vi "Main.vi"() -> ()   [LabVIEW 2019, in "Server.lvlib"]
doc: "This template is based off of the Queued Message Handler design pattern and the Queued Message Handler project template that ships with LabVIEW.\n\nThe main difference is that the queue is private to this module and communication between modules is performed via Broadcast and Request events.\n\nRequest events are wrapped in public API methods and are handled in the Event Handling Loop (EHL) of this VI. Any module can register for Broadcast events sent by this module. The EHL generates messages based on user interface actions.\n\nThe Message Handling Loop (MHL) processes messages generated by the EHL, or by other messages. The messages are string values, so new messages can be added easily to the Message Cases case structure in the MHL. Each message cluster can also provide an optional value for Message Data, which is a variant that can be converted to whatever message-specific data is required.\n_____\nBased on Delacor QMH Project Template 4.2.1.64."
uses:
  Server.lvlib
  <vilib>/Delacor/Delacor QMH/Libraries/Module Admin_class/Delacor_lib_QMH_Module Admin.lvclass
  TypeDef/ISO.ctl
  TypeDef/Link.ctl
  TypeDef/Noise.ctl
  Module Data--cluster.ctl
  Do Something Argument--cluster.ctl
  <vilib>/Delacor/Delacor QMH/Libraries/Message Queue_class/Delacor_lib_QMH_Message Queue.lvclass/Delacor_lib_QMH_Message Queue.ctl
  Do Something Else Argument--cluster.ctl
  Do Something Else and Wait for Reply Argument--cluster.ctl
  Do Something Else and Wait (Reply Payload)--cluster.ctl
  Stop Argument--cluster.ctl
  TypeDef/Sett data.ctl
  Update control Argument--cluster.ctl
  <vilib>/Delacor/Delacor QMH/Libraries/Module Admin_class/Delacor_lib_QMH_Module Admin.lvclass/Delacor_lib_QMH_Module Admin.ctl
  TypeDef/Analys data.ctl
  TypeDef/Analys type.ctl
  <vilib>/Delacor/Delacor QMH/Libraries/Message Queue_class/Delacor_lib_QMH_Enqueue Message (Single).vi
  <vilib>/Delacor/Delacor QMH/Libraries/Module Admin_class/Delacor_lib_QMH_Get External Launch.vi
  <vilib>/Utility/error.llb/Error Cluster From Error Code.vi
  <vilib>/ErrorRing/Error Ring.xnode
  <vilib>/Delacor/Delacor QMH/Libraries/Message Queue_class/Delacor_lib_QMH_Message Queue.lvclass
  Interrogator/DOWNLINK.lvlib
  UPLINK/UPLINK.lvlib
  Setting Panel/Setting Panel.lvlib
panel:
  in  "Tab Control":enum32{"Main", "Setting"}(tab)
  in  "Иммитатор расстояния":dbl(slide)=3.0 min=3.0 max=1500.0 step=1.0 scale=3.0..1500.0
  in  "Усилитель сигнала":dbl(knob)=1.0 min=1.0 max=100.0 step=1.0 scale=1.0..30.0
  in  "Выбор стандарта":T1
  in  "Аттенюатор шума":dbl(knob)=1.0 min=1.0 max=10.0 step=0.1 scale=1.0..30.0
  in  "Bit rate":dbl=32.0 min=4.0 max=128.0 step=4.0
  in  "Filter":i32=3 min=1 max=15 step=1
  in  "Type noise w":T2
  in  "M w":cluster{"Метка":i64, "Считыветель":i64}={"Метка"=10, "Считыветель"=100} {"Считыветель" min=10 max=10 step=100; "Метка" min=10 max=10 step=100}
  in  "BM":cluster{"R":dbl, "C":dbl, "L":dbl}={"R"=1.0, "C"=0.01, "L"=1e-05} {"L" min=1e-05 max=1.5e-05 step=1e-06 format="%#_6p"; "C" min=0.01 max=0.15 step=0.001 format="%#_6p"; "R" min=1.0 max=150.0 step=1.0 format="%#_6p"}
  in  "BI":cluster{"R":dbl, "C":dbl, "L":dbl}={"R"=1.0, "C"=0.01, "L"=1e-05} {"L" min=1e-05 max=1.5e-05 step=1e-06 format="%#_6p"; "C" min=0.01 max=0.15 step=0.001 format="%#_6p"; "R" min=1.0 max=150.0 step=1.0 format="%#_6p"}
  in  "Apply":bool
  in  "Shutdown":bool
  in  "Link":T3
  in  "Simulate MHL Error":bool
  in  "Simulate EHL Error":bool
  out "error out":errorcluster
  in  "Module Admin":refnum<class "Delacor_lib_QMH_Module Admin.lvclass">
  out "X":dbl
  out "Status":string
  in  "Do Something Else <Replace Me>":bool
  in  "Do Something <Replace Me>":bool
  # "Настройки"
  # "мм"
  # "БУПУЭМСС"
  # "БУПУЭМСМ"
  # "Коэффициент модуляции, %"
  # "Порядок фильтра"
  # "Скорость"
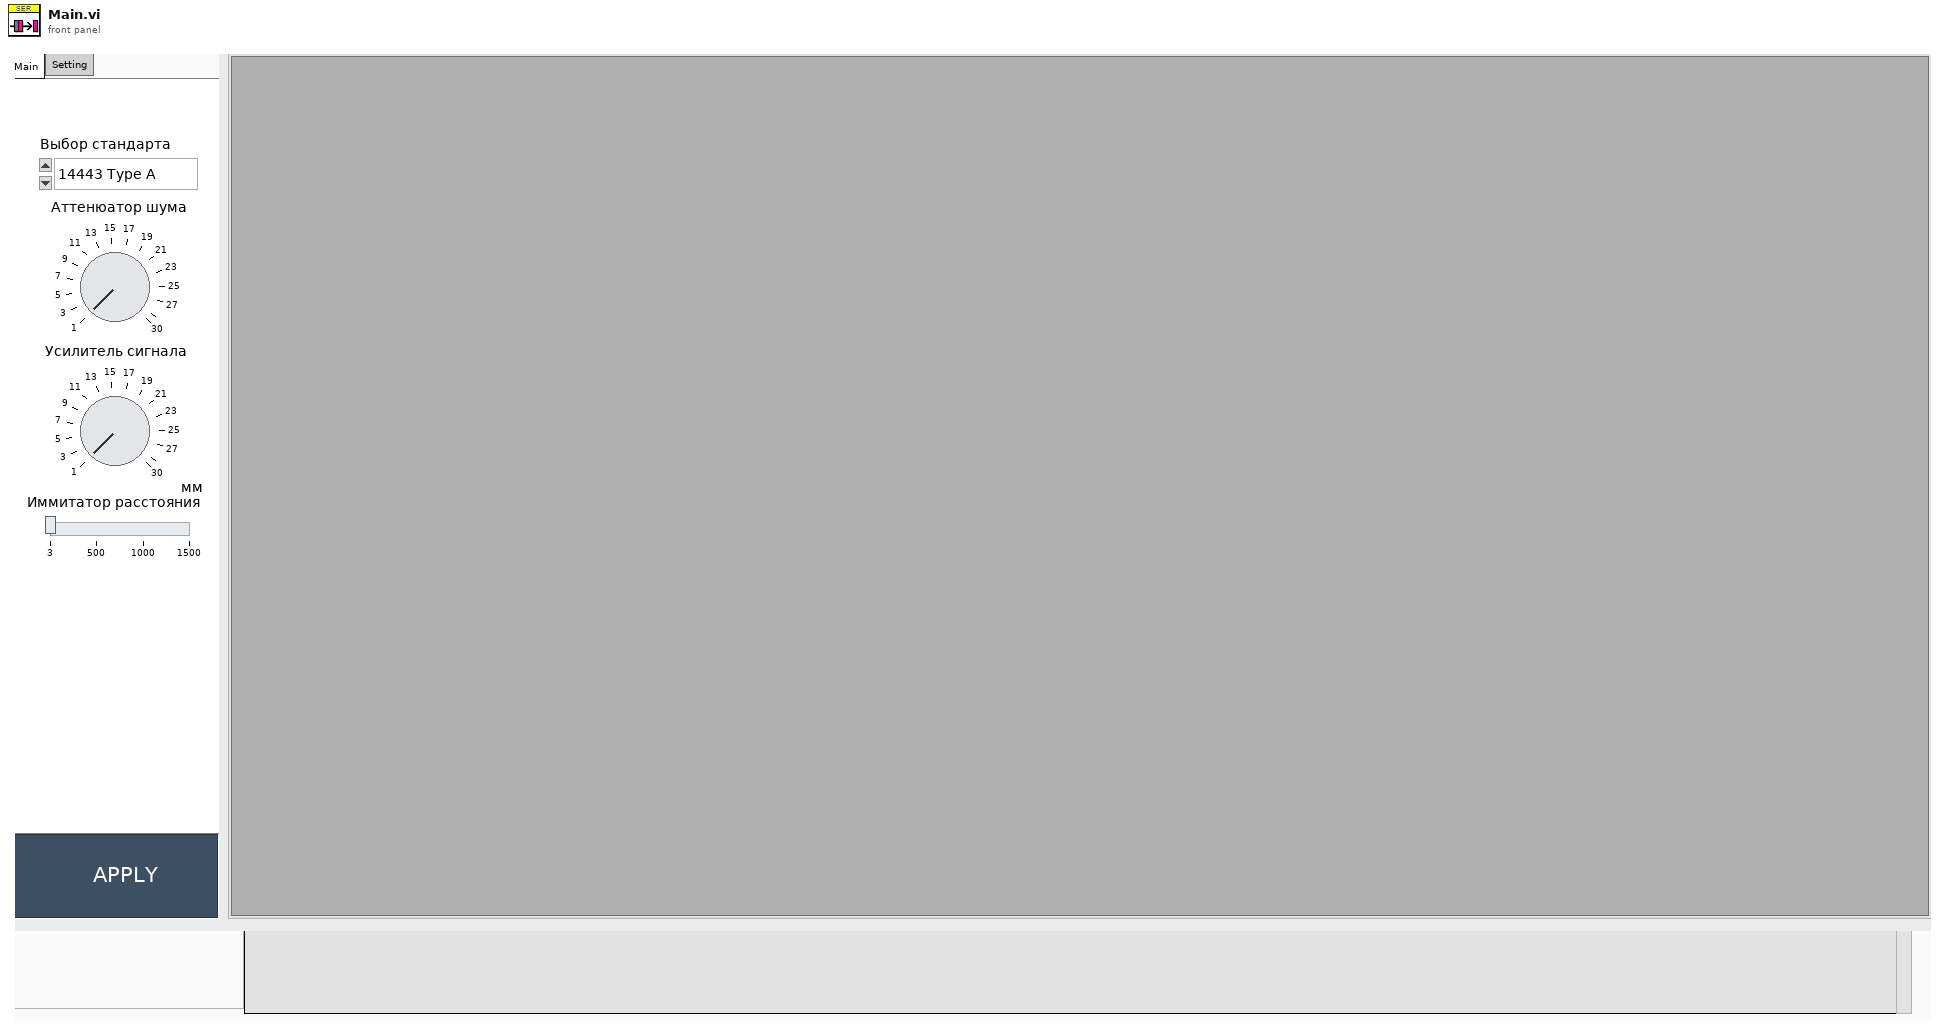
[diagram p1: front panel]
types:
  T1 = typedef "ISO.ctl" = enum16{"14443 Type A", "14443 Type B", "Felica", "15693"}
  T2 = typedef "Noise.ctl" = enum16{"Гауссовский шум", "Белый шум"}
  T3 = typedef "Link.ctl" = enum16{"UPLINK", "DOWNLINK"}
  T4 = typedef "Server.lvlib/Request Events--cluster.ctl" = cluster{"Stop Module":refnum<user-event>, "Do Something":refnum<user-event>, "Do Something Else":refnum<user-event>, "Do Something Else and Wait for Reply":refnum<user-event>, "Show Panel":refnum<user-event>, "Hide Panel":refnum<user-event>, "Get Module Execution Status":refnum<user-event>, "Show Diagram":refnum<user-event>, "Update control":refnum<user-event>}
  T5 = typedef "UPLINK.lvlib/Broadcast Events--cluster.ctl" = cluster{"Module Did Init":refnum<user-event>, "Status Updated":refnum<user-event>, "Error Reported":refnum<user-event>, "Did Something":refnum<user-event>, "Module Did Stop":refnum<user-event>, "Update Module Execution Status":refnum<user-event>}
  T6 = typedef "DOWNLINK.lvlib/Broadcast Events--cluster.ctl" = cluster{"Module Did Init":refnum<user-event>, "Status Updated":refnum<user-event>, "Error Reported":refnum<user-event>, "Did Something":refnum<user-event>, "Module Did Stop":refnum<user-event>, "Update Module Execution Status":refnum<user-event>}
  T7 = typedef "Setting Panel.lvlib/Broadcast Events--cluster.ctl" = cluster{"Module Did Init":refnum<user-event>, "Status Updated":refnum<user-event>, "Error Reported":refnum<user-event>, "Did Something":refnum<user-event>, "Module Did Stop":refnum<user-event>, "Update Module Execution Status":refnum<user-event>, "Get data":refnum<user-event>}
  T8 = typedef "Server.lvlib/Module Data--cluster.ctl" = cluster{"Status":string}
  T9 = typedef "Server.lvlib/Do Something Argument--cluster.ctl" = cluster{"Do Something Msg":string}
  T10 = typedef "Server.lvlib/Do Something Else Argument--cluster.ctl" = cluster{"Do Something Else Msg":string, "X":dbl}
  T11 = typedef "Server.lvlib/Do Something Else and Wait for Reply Argument--cluster.ctl" = cluster{"Do Something Else Msg":string, "X":dbl, "Wait Notifier":refnum<notifier>, "wait for reply":bool}
  T12 = enum32{"invalid lock state", "Not Locked", "Locked (No Password)", "Password-protected"}
  T13 = typedef "Server.lvlib/Stop Argument--cluster.ctl" = cluster{"Origin":string, "Exit via Stop Module Req?":bool, "Wait for Module to stop?":bool}
  T14 = typedef "Sett data.ctl" = cluster{"Filter":i32, "Gain":dbl, "Bit rate":dbl, "ISO/IEC w ":T1, "BI":cluster{"R":dbl, "C":dbl, "L":dbl}, "BM":cluster{"R":dbl, "C":dbl, "L":dbl}, "M":cluster{"Метка":i64, "Считыветель":i64}, "Type noise":T2, "Link":T3, "Noise attenuator":dbl, "Signal gain":dbl, "Distance":dbl}
  T15 = enum8{"Enabled", "Disabled", "Disabled and Grayed Out"}
  T16 = typedef "Server.lvlib/Update control Argument--cluster.ctl" = cluster{"Variant":variant}
  T17 = enum32{"Invalid", "Standard", "Closed", "Hidden", "Minimized", "Maximized"}
  T18 = typedef "Server.lvlib/Do Something Else and Wait (Reply Payload)--cluster.ctl" = cluster{"Value":dbl, "error":errorcluster}
  T19 = typedef "Analys data.ctl" = cluster{"min attenuator":dbl, "max distanse":dbl, "num sample":dbl, "type":T20}
  T20 = typedef "Analys type.ctl" = enum16{"Noise", "Distance"}
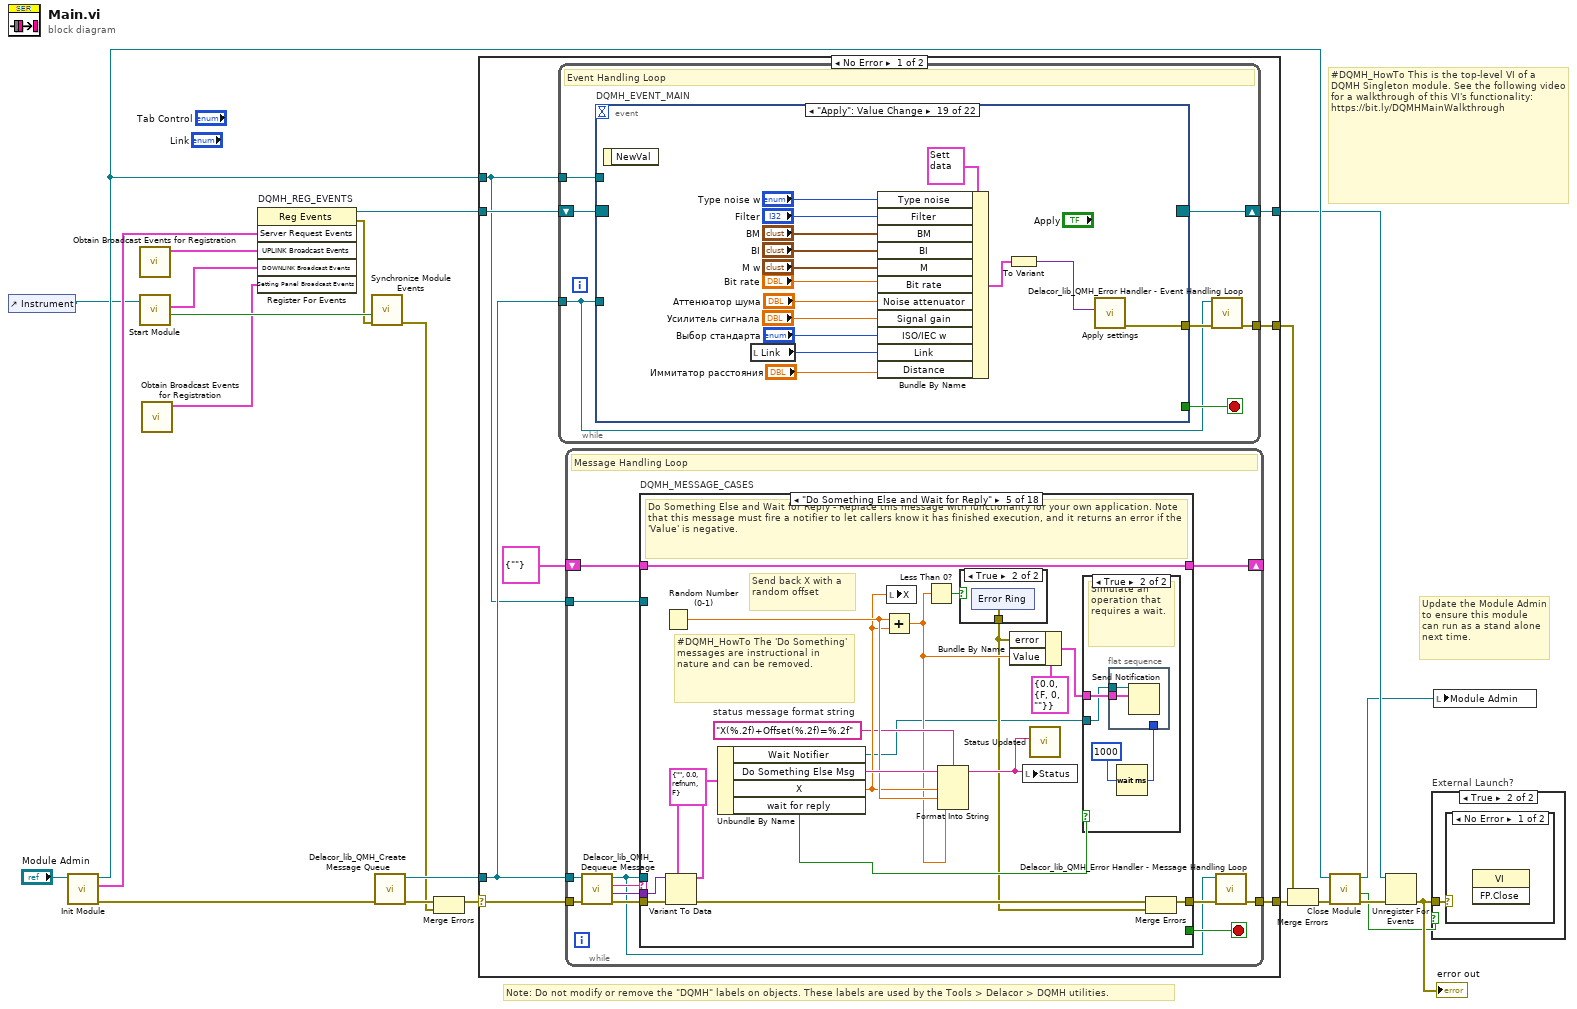
[diagram p0: block diagram]
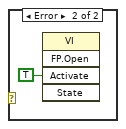
[diagram p3: hidden frame]
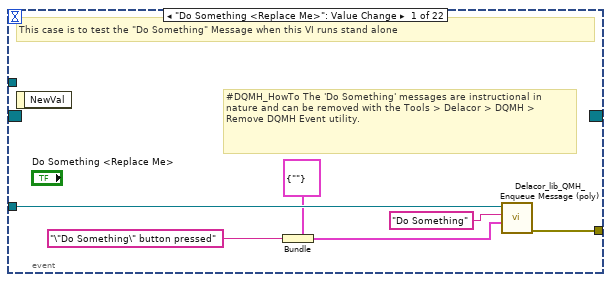
[diagram p4: hidden frame]
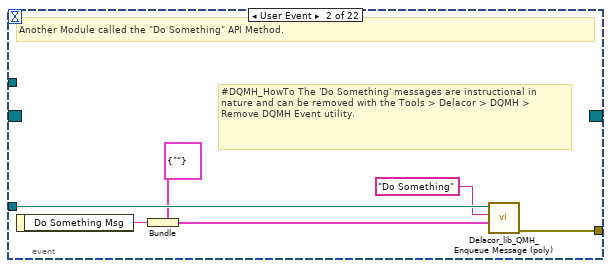
[diagram p5: hidden frame]
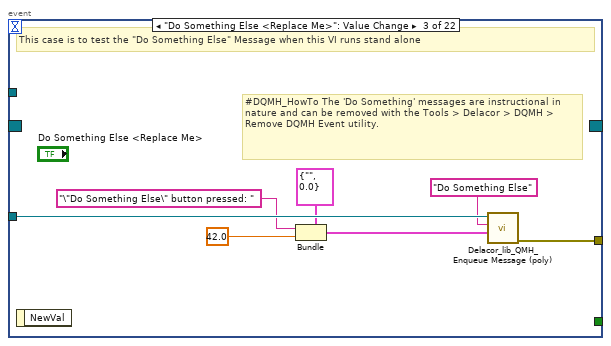
[diagram p6: hidden frame]
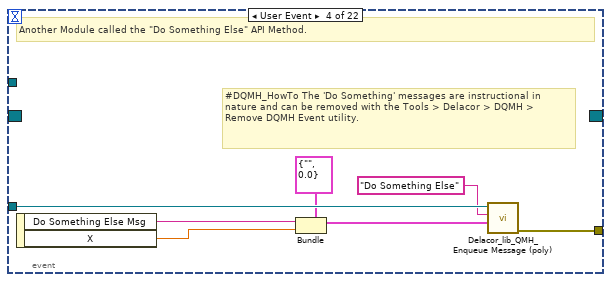
[diagram p7: hidden frame]
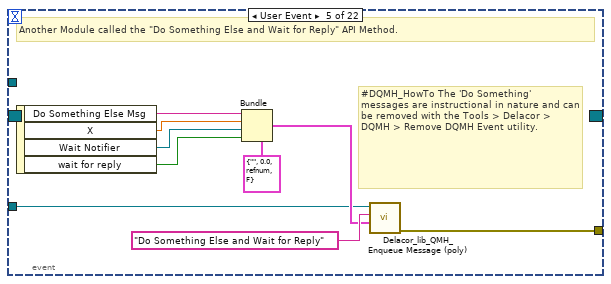
[diagram p8: hidden frame]
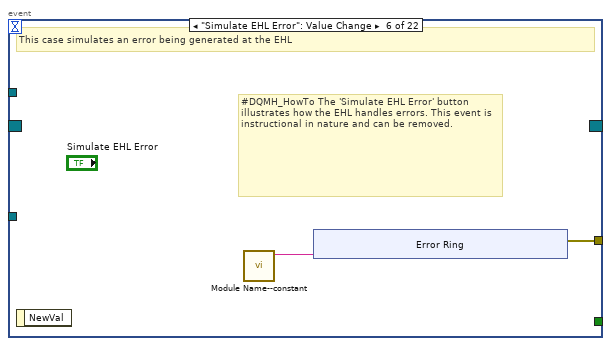
[diagram p9: hidden frame]
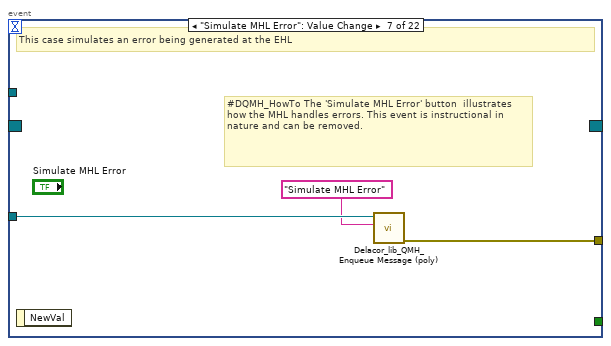
[diagram p10: hidden frame]
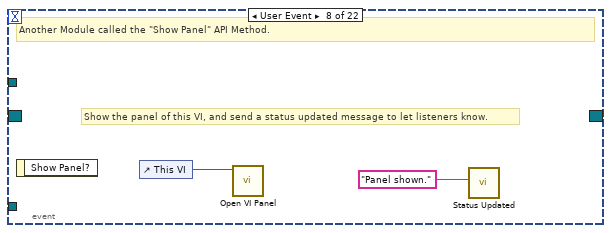
[diagram p11: hidden frame]
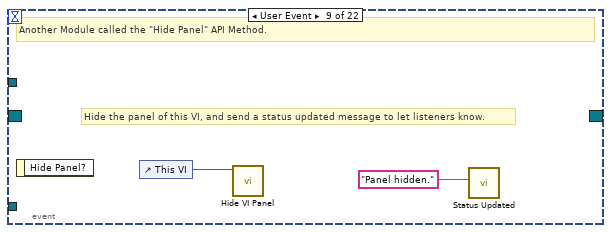
[diagram p12: hidden frame]
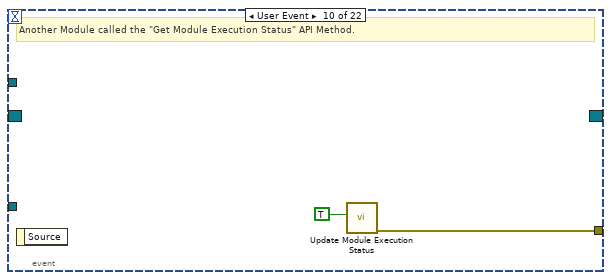
[diagram p13: hidden frame]
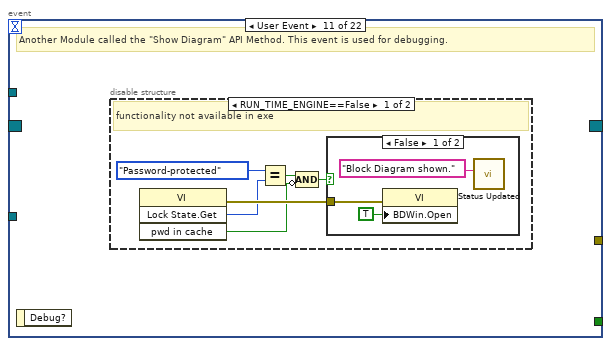
[diagram p14: hidden frame]
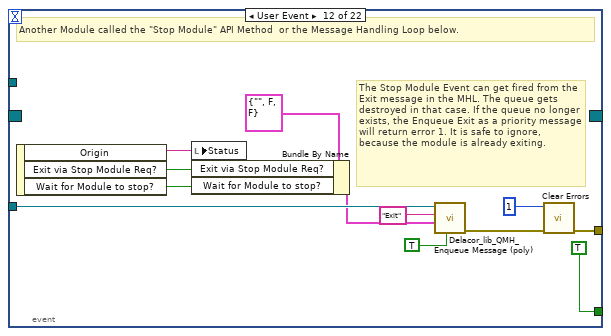
[diagram p17: hidden frame]
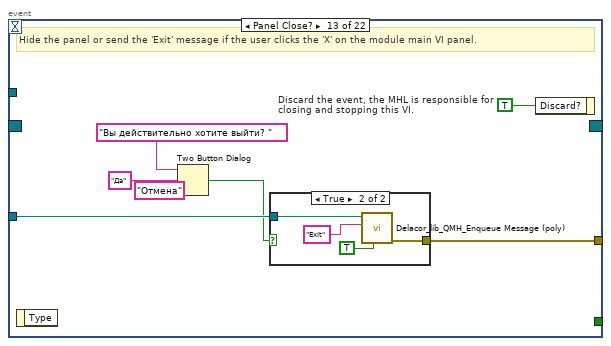
[diagram p18: hidden frame]
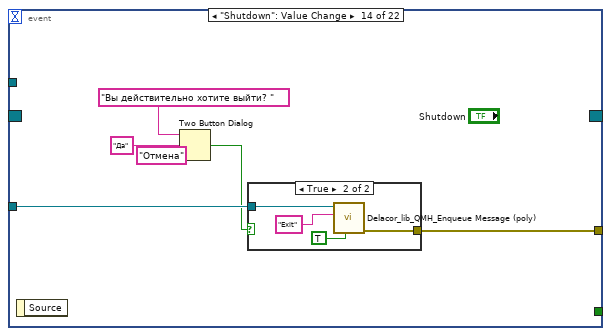
[diagram p20: hidden frame]
diagram:
  # "#DQMH_HowTo This is the top-level VI of a DQMH Singleton module. See the following video for a walkthrough of this VI's functionality: https://bit.ly/DQMHMainWalkthrough"
  # "Note: Do not modify or remove the \"DQMH\" labels on objects. These labels are used by the Tools > Delacor > DQMH utilities."
  # "Update the Module Admin to ensure this module can run as a stand alone next time."
  n1 = control-ref of="Instrument"() -> (w2:refnum<vi>)
  n2 = call "Init Module.vi"("Singleton Module Admin in"="Module Admin") -> ("error out"=w22:errorcluster, "Server Request Events"=w12:T4, "Singleton Module Admin out"=w15:refnum<class "Delacor_lib_QMH_Module Admin.lvclass">)  [unwired: 8 in]
  n3 = call "Obtain Broadcast Events for Registration.vi"() -> ("UPLINK Broadcast Events"=w7:T5)  [unwired: 9 in, 2 out]
  n4 = call "Start Module.vi"("Subpanel Ref"=w2) -> ("Wait for Event Sync?"=w5:bool, "DOWNLINK Broadcast Events"=w6:T6)  [unwired: 7 in, 2 out]
  n5 = call "Obtain Broadcast Events for Registration.vi"() -> ("Setting Panel Broadcast Events"=w1:T7)  [unwired: 9 in, 2 out]
  n6 = register-events "DQMH_REG_EVENTS"(w12, w7, w6, w1) -> (reference out=w13:refnum<event-registration>, error out=w4:errorcluster)  [unwired: 2 in]
  n7 = call "Synchronize Module Events.vi"("error in (no error)"=w4, "Wait for Event Sync?"=w5) -> ("error out"=w3:errorcluster)  [unwired: 9 in]
  n8 = call <vilib>:"Delacor_lib_QMH_Create Message Queue.vi"("error in (no error)"=w22) -> ("error out"=w17:errorcluster, "Message Queue"=w11:refnum<class "Delacor_lib_QMH_Message Queue.lvclass">)  [unwired: 9 in]
  n9 = Merge Errors(w17, w3) -> (w16:errorcluster)
  n10 = case shown="No Error" w16 {
    selector: w16 -> [w29 w511]
    tunnel: [w31 w511] -> w23
    tunnel: [w28 w508] -> w14
    tunnel: w13 -> [w26 w508]
    tunnel: w11 -> [w25 _]
    tunnel: [w30 _] -> w20
    tunnel: w15 -> [w24 w504]
    frame No Error {
      n11 = while {
        tunnel: w25 -> [w32]
        shift-right: [w35] -> w28
        shift-left: w26 -> [w36]
        tunnel: [w37] -> w30
        tunnel: w24 -> [w33]
        stop <- w34 stop-if-true
        # "Event Handling Loop"
        n12 = event "DQMH_EVENT_MAIN" shown="[18] \"Apply\": Value Change" {
          selector: w36 -> [_ _ _ _ _ _ _ _ _ _ _ _ _ _ w136 _ _ _ _ _ _ _]
          dyn-events: [_ _ _ _ _ _ _ _ _ _ _ _ _ _ _ _ _ _ _ _ _ _] -> w35
          timeout: _ -> [_ _ _ _ _ _ _ _ _ _ _ _ _ _ _ _ _ _ _ _ _ _]
          tunnel: [_ _ _ _ _ _ _ _ _ _ _ TRUE ("Discard?") _ _ _ _ _ _ _ _ _ _] -> w34
          tunnel: w32 -> [w43 w49 w56 w63 w66 _ w84 _ _ _ _ w108 w117 w129 _ _ _ w156 _ w177 w203 w209]
          tunnel: [w44 w50 w57 w64 w73 w75 w85 _ _ w91 _ w111 w119 w128 _ _ _ w155 w172 w173 w202 w204] -> w38
          tunnel: w33 -> [_ _ _ _ _ _ _ _ _ _ _ _ _ _ _ _ _ _ _ _ _ _]
          event "Do Something <Replace Me>": Value Change {
            # "#DQMH_HowTo The 'Do Something' messages are instructional in nature and can be removed with the Tools > Delacor > DQMH > Remove DQMH Event utility."
            # "This case is to test the \"Do Something\" Message when this VI runs stand alone"
            n13 = event-data() -> ()  [unwired: 1 in, 1 out]
            n14 = Bundle(cluster=T9 {"Do Something Msg"=""} ("Do Something Argument"), "Do Something Msg"="\"Do Something\" button pressed" ("\"Do Something\" button pressed")) -> (w39:T9)
            n15 = call-poly <vilib>:"Delacor_lib_QMH_Enqueue Message (poly).vi"("Message Data"=w39, "Message"="Do Something", "Message Queue in"=w43) -> ("error out"=w44:errorcluster)  [unwired: 7 in, 1 out]
          }
          event User Event {
            # "#DQMH_HowTo The 'Do Something' messages are instructional in nature and can be removed with the Tools > Delacor > DQMH > Remove DQMH Event utility."
            # "Another Module called the \"Do Something\" API Method."
            n16 = event-data() -> ("Do Something Msg"=w46:string)  [unwired: 1 in]
            n17 = Bundle(cluster=T9 {"Do Something Msg"=""} ("Do Something Argument"), "Do Something Msg"=w46) -> (w45:T9)
            n18 = call-poly <vilib>:"Delacor_lib_QMH_Enqueue Message (poly).vi"("Message Data"=w45, "Message"="Do Something", "Message Queue in"=w49) -> ("error out"=w50:errorcluster)  [unwired: 7 in, 1 out]
          }
          event "Do Something Else <Replace Me>": Value Change {
            # "#DQMH_HowTo The 'Do Something' messages are instructional in nature and can be removed with the Tools > Delacor > DQMH > Remove DQMH Event utility."
            # "This case is to test the \"Do Something Else\" Message when this VI runs stand alone"
            n19 = event-data() -> ()  [unwired: 1 in, 1 out]
            n20 = Bundle(cluster=T10 {"Do Something Else Msg"="", "X"=0.0} ("Do Something Else Argument"), "Do Something Else Msg"="\"Do Something Else\" button pressed: " ("\"Do Something Else\" button pressed"), "X"=42.0) -> (w53:T10)
            n21 = call-poly <vilib>:"Delacor_lib_QMH_Enqueue Message (poly).vi"("Message Data"=w53, "Message"="Do Something Else", "Message Queue in"=w56) -> ("error out"=w57:errorcluster)  [unwired: 7 in, 1 out]
          }
          event User Event {
            # "#DQMH_HowTo The 'Do Something' messages are instructional in nature and can be removed with the Tools > Delacor > DQMH > Remove DQMH Event utility."
            # "Another Module called the \"Do Something Else\" API Method."
            n22 = event-data() -> ("Do Something Else Msg"=w59:string, "X"=w58:dbl)  [unwired: 1 in]
            n23 = Bundle(cluster=T10 {"Do Something Else Msg"="", "X"=0.0} ("Do Something Else Argument"), "Do Something Else Msg"=w59, "X"=w58) -> (w60:T10)
            n24 = call-poly <vilib>:"Delacor_lib_QMH_Enqueue Message (poly).vi"("Message Data"=w60, "Message"="Do Something Else", "Message Queue in"=w63) -> ("error out"=w64:errorcluster)  [unwired: 7 in, 1 out]
          }
          event User Event {
            # "#DQMH_HowTo The 'Do Something' messages are instructional in nature and can be removed with the Tools > Delacor > DQMH > Remove DQMH Event utility."
            # "Another Module called the \"Do Something Else and Wait for Reply\" API Method."
            n25 = event-data() -> ("Do Something Else Msg"=w69:string, "X"=w68:dbl, "Wait Notifier"=w67:refnum<notifier>, "wait for reply"=w65:bool)  [unwired: 1 in]
            n26 = Bundle(cluster=T11 {"Do Something Else Msg"="", "X"=0.0, "Wait Notifier"=refnum, "wait for reply"=FALSE} ("Do Something Else and Wait for Reply Argument"), "Do Something Else Msg"=w69, "X"=w68, "Wait Notifier"=w67, "wait for reply"=w65) -> (w70:T11)
            n27 = call-poly <vilib>:"Delacor_lib_QMH_Enqueue Message (poly).vi"("Message Data"=w70, "Message"="Do Something Else and Wait for Reply", "Message Queue in"=w66) -> ("error out"=w73:errorcluster)  [unwired: 7 in, 1 out]
          }
          event "Simulate EHL Error": Value Change {
            # "#DQMH_HowTo The 'Simulate EHL Error' button  illustrates how the EHL handles errors. This event is instructional in nature and can be removed."
            # "This case simulates an error being generated at the EHL"
            n28 = event-data() -> ()  [unwired: 1 in, 1 out]
            n29 = call "Module Name--constant.vi"() -> ("Module Name"=w74:string)  [unwired: 11 in]
            n30 = xnode "Error Ring"("parameter 0"=w74) -> ("error out"=w75:errorcluster)
          }
          event "Simulate MHL Error": Value Change {
            # "#DQMH_HowTo The 'Simulate MHL Error' button  illustrates how the MHL handles errors. This event is instructional in nature and can be removed."
            # "This case simulates an error being generated at the EHL"
            n31 = event-data() -> ()  [unwired: 1 in, 1 out]
            n32 = call-poly <vilib>:"Delacor_lib_QMH_Enqueue Message (poly).vi"("Message"="Simulate MHL Error", "Message Queue in"=w84) -> ("error out"=w85:errorcluster)  [unwired: 8 in, 1 out]
          }
          event User Event {
            # "Show the panel of this VI, and send a status updated message to let listeners know."
            # "Another Module called the \"Show Panel\" API Method."
            n33 = event-data() -> ()  [unwired: 1 in, 1 out]
            n34 = control-ref of="This VI"() -> (w87:refnum<vi>)
            n35 = call "Open VI Panel.vi"("VI"=w87) -> ()  [unwired: 10 in, 1 out]
            n36 = call "Status Updated.vi"("Status"="Panel shown." ("format string")) -> ()  [unwired: 10 in, 1 out]
          }
          event User Event {
            # "Hide the panel of this VI, and send a status updated message to let listeners know."
            # "Another Module called the \"Hide Panel\" API Method."
            n37 = event-data() -> ()  [unwired: 1 in, 1 out]
            n38 = control-ref of="This VI"() -> (w89:refnum<vi>)
            n39 = call "Hide VI Panel.vi"("VI"=w89) -> ()  [unwired: 10 in, 1 out]
            n40 = call "Status Updated.vi"("Status"="Panel hidden." ("format string")) -> ()  [unwired: 10 in, 1 out]
          }
          event User Event {
            # "Another Module called the \"Get Module Execution Status\" API Method."
            n41 = event-data() -> ()  [unwired: 1 in, 1 out]
            n42 = call "Update Module Execution Status.vi"("Running?"=TRUE) -> ("error out"=w91:errorcluster)  [unwired: 10 in]
          }
          event User Event {
            # "Another Module called the \"Show Diagram\" API Method. This event is used for debugging."
            n43 = event-data() -> ()  [unwired: 1 in, 1 out]
            n44 = disable-structure shown="RUN_TIME_ENGINE==False" {
              frame condition #0 (active) {
                # "functionality not available in exe"
                n45 = invoke class="VI" method="Lock State.Get"() -> (error out=w97:errorcluster, "Get Lock State"=w96:T12, "pwd in cache"=w93:bool)  [unwired: 4 in, 1 out]
                n46 = Equal?(x=T12."Password-protected", y=w96) -> (x = y?=w94:bool)
                n47 = Compound Arithmetic op=AND(w94, invert w93) -> (w92:bool)
                n48 = case shown="False" w92 {
                  tunnel: w97 -> [w100 _]
                  frame False {
                    n49 = property class="VI"(error in=w100, "BDWin.Open"=TRUE ("Block Diagram Window:Open")) -> ()  [unwired: 1 in, 2 out]
                    n50 = call "Status Updated.vi"("Status"="Block Diagram shown." ("format string")) -> ()  [unwired: 10 in, 1 out]
                  }
                  frame True {
                    # "Password-protected VI, and the password is not in the cache. Do not show the diagram."
                  }
                }
              }
              frame condition #1 {
              }
            }
          }
          event User Event {
            # "The Stop Module Event can get fired from the Exit message in the MHL. The queue gets destroyed in that case. If the queue no longer exists, the Enqueue Exit as a priority message will return error 1. It is safe to ignore, because the module is already exiting."
            # "Another Module called the \"Stop Module\" API Method  or the Message Handling Loop below."
            n51 = event-data() -> ("Origin"=w107:string, "Exit via Stop Module Req?"=w103:bool, "Wait for Module to stop?"=w102:bool)  [unwired: 1 in]
            n52 = local write "Status"(w107) -> ()
            n53 = Bundle By Name(cluster=T13 {"Origin"="", "Exit via Stop Module Req?"=FALSE, "Wait for Module to stop?"=FALSE} ("Stop Argument"), "Exit via Stop Module Req?"=w103, "Wait for Module to stop?"=w102) -> (w101:T13)
            n54 = call-poly <vilib>:"Delacor_lib_QMH_Enqueue Message (poly).vi"("Priority Message? (F)"=TRUE, "Message Data"=w101, "Message"="Exit", "Message Queue in"=w108) -> ("error out"=w112:errorcluster)  [unwired: 6 in, 1 out]
            n55 = call <vilib>:"Clear Errors.vi"("error in (no error)"=w112, "specific error code to clear (0: all)"=1) -> ("error out"=w111:errorcluster)  [unwired: 4 in, 1 out]
          }
          event Panel Close? {
            w118 = TRUE  # Discard the event, the MHL is responsible for closing and stopping this VI.
            # "Hide the panel or send the 'Exit' message if the user clicks the 'X' on the module main VI panel."
            n56 = event-data() -> ()  [unwired: 1 in, 1 out]
            n57 = Two Button Dialog(message="Вы действительно хотите выйти? ", 1:"Отмена" ("F button name (\"Cancel\")"), 2:"Да" ("T button name (\"OK\")")) -> (T button?=w113:bool)
            n58 = case shown="True" w113 {
              tunnel: [_ w123] -> w119
              tunnel: w117 -> [_ w122]
              frame False {
              }
              frame True {
                n59 = call-poly <vilib>:"Delacor_lib_QMH_Enqueue Message (poly).vi"("Priority Message? (F)"=TRUE, "Message"="Exit", "Message Queue in"=w122) -> ("error out"=w123:errorcluster)  [unwired: 7 in, 1 out]
              }
            }
            n60 = event-data("Discard?"=w118) -> ()  [unwired: 1 in, 1 out]
          }
          event "Shutdown": Value Change {
            n61 = event-data() -> ()  [unwired: 1 in, 1 out]
            n62 = Two Button Dialog(message="Вы действительно хотите выйти? ", 1:"Отмена" ("F button name (\"Cancel\")"), 2:"Да" ("T button name (\"OK\")")) -> (T button?=w124:bool)
            n63 = case shown="True" w124 {
              tunnel: w129 -> [_ w131]
              tunnel: [_ w130] -> w128
              frame False {
              }
              frame True {
                n64 = call-poly <vilib>:"Delacor_lib_QMH_Enqueue Message (poly).vi"("Priority Message? (F)"=TRUE, "Message"="Exit", "Message Queue in"=w131) -> ("error out"=w130:errorcluster)  [unwired: 7 in, 1 out]
              }
            }
          }
          event User Event {
            n65 = event-data() -> ()  [unwired: 1 in, 1 out]
            n66 = call "Start Module.vi"() -> ("error out"=w144:errorcluster, "Wait for Event Sync?"=w143:bool, "UPLINK Broadcast Events"=w134:T5)  [unwired: 8 in, 1 out]
            n67 = call "Start Module.vi"() -> ("error out"=w142:errorcluster, "Wait for Event Sync?"=w141:bool, "Setting Panel Broadcast Events"=w135:T7)  [unwired: 8 in, 1 out]
            n68 = call "Synchronize Module Events.vi"("error in (no error)"=w144, "Wait for Event Sync?"=w143) -> ()  [unwired: 9 in, 1 out]
            n69 = call "Synchronize Module Events.vi"("error in (no error)"=w142, "Wait for Event Sync?"=w141) -> ()  [unwired: 9 in, 1 out]
            n70 = register-events(reference=w136, w134, w135) -> ()  [unwired: 3 in, 2 out]
            n71 = local read "Status"() -> (w140:string)
            n72 = Concatenate Strings("Запуск всех модулей" ("format string"), "\r", w140) -> (w139:string)
            n73 = local write "Status"(w139) -> ()
          }
          event User Event {
            n74 = event-data() -> ("Status"=w146:string)  [unwired: 1 in]
            n75 = local read "Status"() -> (w147:string)
            n76 = Concatenate Strings(w146, "\r", w147) -> (w145:string)
            n77 = local write "Status"(w145) -> ()
          }
          event User Event {
            n78 = event-data() -> ("Status"=w150:string)  [unwired: 1 in]
            n79 = local read "Status"() -> (w151:string)
            n80 = Concatenate Strings(w150, "\r", w151) -> (w149:string)
            n81 = local write "Status"(w149) -> ()
          }
          event Menu Selection (User) {
            n82 = event-data() -> ("ItemTag"=w154:string)  [unwired: 1 in]
            n83 = To Variant(anything=w154) -> (Variant=w153:variant)
            n84 = call-poly <vilib>:"Delacor_lib_QMH_Enqueue Message (poly).vi"("Message Data"=w153, "Message"="USER menu", "Message Queue in"=w156) -> ("error out"=w155:errorcluster)  [unwired: 7 in, 1 out]
          }
          event "Apply": Value Change {
            n85 = event-data() -> ()  [unwired: 1 in, 1 out]
            n86 = local read "Link"() -> (w168:T3)
            n87 = Bundle By Name(cluster=T14 {"Filter"=0, "Gain"=0.0, "Bit rate"=0.0, "ISO/IEC w "=enum."14443 Type A", "BI"={"R"=0.0, "C"=0.0, "L"=0.0}, "BM"={"R"=0.0, "C"=0.0, "L"=0.0}, "M"={"Метка"=4, "Считыветель"=4}, "Type noise"=enum."Гауссовский шум", "Link"=enum."UPLINK", "Noise attenuator"=0.0, "Signal gain"=1.0, "Distance"=0.0} ("Sett data"), "Type noise"="Type noise w", "Filter"="Filter", "BM"="BM", "BI"="BI", "M"="M w", "Bit rate"="Bit rate", "Noise attenuator"="Аттенюатор шума", "Signal gain"="Усилитель сигнала", "ISO/IEC w"="Выбор стандарта", "Link"=w168, "Distance"="Иммитатор расстояния") -> (w165:T14)
            n88 = To Variant(anything=w165) -> (Variant=w166:variant)
            n89 = call "Apply settings.vi"("Data"=w166) -> ("error out"=w172:errorcluster)  [unwired: 10 in]
          }
          event Value Change {
            w181 = T1[] [enum."Felica", enum."15693"] items=["14443 Type A", "14443 Type B", "Felica", "15693"]
            n90 = event-data() -> ("CtlRef"=w189:refnum<vi>, "OldVal"=w187:T1, "NewVal"=w176:T1)  [unwired: 1 in]
            n91 = call-poly <vilib>:"Delacor_lib_QMH_Enqueue Message (poly).vi"("Message Data"=w176, "Message"="Read ini", "Message Queue in"=w177) -> ("error out"=w174:errorcluster)  [unwired: 7 in, 1 out]
            n92 = for {
              tunnel: w181 -> [w199] mode=indexing
              shift-right: [w195] -> w178
              shift-left: FALSE -> [w196]
              tunnel: w176 -> [w198]
              n93 = Equal?(x=w199, y=w198) -> (x = y?=w197:bool)
              n94 = Or(x=w196, y=w197) -> (x .or. y?=w195:bool)
            }
            n95 = property class="Enum (strict)"(reference=w189) -> ("Strings []"=w188:string[])  [unwired: 1 in, 2 out]
            n96 = case shown="True" w178 {
              tunnel: [T15."Enabled" ("Disabled") T15."Disabled and Grayed Out" ("Disabled")] -> w179
              frame False {
              }
              frame True {
              }
            }
            n97 = Index Array(array=w188, index #1=w187, index #2=w176) -> (element #1=w185:string, element #2=w184:string)
            n98 = local read "Status"() -> (w191:string)
            n99 = control-ref of="Apply"() -> (w182:refnum<vi>)
            n100 = Format Into String(format string="Смена стандарта:%1s -> %2s" ("string"), error in=w174, w185, w184) -> (resulting string=w183:string, error out=w173:errorcluster)  [unwired: 1 in]
            n101 = Concatenate Strings(w183, "\r", w191) -> (w190:string)
            n102 = property class="Bool"(reference=w182, "DisabledEnum"=w179) -> ()  [unwired: 1 in, 2 out]
            n103 = local write "Status"(w190) -> ()
          }
          event User Event {
            n104 = event-data() -> ("Variant"=w201:variant)  [unwired: 1 in]
            n105 = call-poly <vilib>:"Delacor_lib_QMH_Enqueue Message (poly).vi"("Message Data"=w201, "Message"="Update control", "Message Queue in"=w203) -> ("error out"=w202:errorcluster)  [unwired: 7 in, 1 out]
          }
          event User Event {
            # "Another Module called the \"Update control\" API Method."
            n106 = event-data() -> ("Variant"=w205:variant)  [unwired: 1 in]
            n107 = Bundle(cluster=T16 {"Variant"=variant} ("Update control Argument"), "Variant"=w205) -> (w206:T16)
            n108 = call-poly <vilib>:"Delacor_lib_QMH_Enqueue Message (poly).vi"("Message Data"=w206, "Message"="Update control BC", "Message Queue in"=w209) -> ("error out"=w204:errorcluster)  [unwired: 7 in, 1 out]
          }
        }
        n109 = call-dynamic "Delacor_lib_QMH_Error Handler - Event Handling Loop.vi"("error in (no error)"=w38, "Message Queue in"=w32) -> ("dup error in"=w37:errorcluster)  [unwired: 8 in, 1 out]
      }
      n110 = while {
        tunnel: w25 -> [w212]
        shift-right: [w216] -> _
        shift-left: T8 {"Status"=""} ("Data Cluster") -> [w217]
        tunnel: w29 -> [w220]
        tunnel: [w218] -> w31
        tunnel: w24 -> [w210]
        stop <- w215 stop-if-true
        # "Message Handling Loop"
        n111 = call-dynamic "Delacor_lib_QMH_Dequeue Message.vi"("error in (no error)"=w220, "Message Queue in"=w212) -> ("error out"=w219:errorcluster, "Message Data"=w213:variant, "Message"=w214:string, "Message Queue out"=w211:refnum<class "Delacor_lib_QMH_Message Queue.lvclass">)  [unwired: 6 in]
        n112 = case "DQMH_MESSAGE_CASES" shown="\"Do Something Else and Wait for Reply\"" w214 {
          selector: w214 -> [_ _ _ _ _ _ _ _ _ _ _ _ _ _ _ _ _ w491]
          tunnel: w211 -> [_ _ _ _ _ _ _ w312 _ _ _ _ _ _ _ w455 w484 _]
          tunnel: w219 -> [w242 w246 w254 w263 w282 w308 w311 w318 w397 w410 w412 w420 w433 w440 w445 w462 w489 w493]
          tunnel: [w240 w246 w252 w262 w281 w306 w310 w320 w399 w410 w411 w419 w434 w440 w444 w458 w486 w494] -> w221
          tunnel: w217 -> [w232 w245 w251 w261 w279 w307 w309 w319 w398 w409 w413 w421 w438 w439 w442 w457 w483 w492]
          tunnel: [w231 w245 w251 w261 w279 w307 w309 w319 w398 w409 w413 w421 w438 w439 w442 w457 w483 w492] -> w216
          tunnel: [_ _ _ _ _ _ _ _ _ _ _ _ _ _ _ _ w482 _] -> w215
          tunnel: w213 -> [_ _ w250 w258 w276 w305 _ w317 w396 _ _ w418 w430 _ _ w456 w481 _]
          tunnel: w210 -> [w233 _ _ _ _ _ _ _ _ _ _ _ _ _ _ w454 w476 _]
          frame "Initialize" {
            w227 = "Зупуск эмулятора" ("Initial Message")
            # "Initialize - Any operation that needs to be done before the module can receive messages. Synchronize Caller Events.vi will inform Start Module.vi that the module has launched and is ready to receive messages. Module Did Init.vi will broadcast that the module initialized."
            n113 = call "Synchronize Caller Events.vi"("error in (no error)"=w242, "Singleton Module Admin in"=w233) -> ("error out"=w241:errorcluster, "Singleton Module Admin out"=w228:refnum<class "Delacor_lib_QMH_Module Admin.lvclass">)  [unwired: 8 in]
            n114 = property class="Module Admin"(reference=w228) -> ("Accessors:External Launch"=w237:bool)  [unwired: 1 in, 2 out]
            n115 = local write "Выбор стандарта"(ISO."14443 Type A" ("Выбор стандарта")) -> ()
            n116 = local write "Иммитатор расстояния"(3.0 ("Иммитатор расстояния")) -> ()
            n117 = local write "Аттенюатор шума"(16.0 ("Noise attenuator")) -> ()
            n118 = local write "Link"(Link."DOWNLINK" ("Link")) -> ()
            n119 = Select(t=T17."Hidden" ("State"), s=w237, f=T17."Standard" ("State")) -> (s? t:f=w234:T17)
            n120 = property class="VI"("Front Panel.Title"="RFID Emulator" ("Front Panel Window:Title")) -> (reference out=w239:refnum<vi>, error out=w244:errorcluster)  [unwired: 2 in]
            n121 = call "Module Name--constant.vi"() -> ("Module Name"=w229:string)  [unwired: 11 in]
            n122 = invoke class="VI" method="FP.Open"(reference=w239, error in=w244, "State"=w234) -> (reference out=w238:refnum<vi>, error out=w243:errorcluster)  [unwired: 2 in, 3 out]
            n123 = Bundle By Name(cluster=w232, "Status"=w227) -> (w231:T8)
            n124 = call "Module Did Init.vi"("error in (no error)"=w241, "Initialized?"=TRUE, "Origin"=w229) -> ("error out"=w240:errorcluster)  [unwired: 8 in]
            n125 = invoke class="VI" method="FP.Center"(reference=w238, error in=w243) -> ()  [unwired: 1 in, 3 out]
            "Status" <- w227
          }
          frame "--- Module Specific ---" {
            # "Separator -- The following cases handle messages specific to this Module."
          }
          frame "Do Something" {
            # "#DQMH_HowTo The 'Do Something' messages are instructional in nature and can be removed with the Tools > Delacor > DQMH > Remove DQMH Event utility."
            # "Do Something - Replace this message with functionality for your own application. Note that this message also fires the \"Did Something\" broadcast event."
            n126 = Variant To Data(error in=w254, type=T9 {"Do Something Msg"=""} ("Do Something Argument"), Variant=w250) -> (data=w249:T9, error out=w253:errorcluster)
            n127 = Unbundle By Name(w249) -> ("Do Something Msg"=w247:string)
            n128 = call "Did Something.vi"("error in (no error)"=w253, "Did Something Msg"=w247) -> ("error out"=w252:errorcluster)  [unwired: 9 in]
            n129 = local write "Status"(w247) -> ()
            n130 = call "Status Updated.vi"("Status"=w247) -> ()  [unwired: 10 in, 1 out]
          }
          frame "Do Something Else" {
            # "#DQMH_HowTo The 'Do Something' messages are instructional in nature and can be removed with the Tools > Delacor > DQMH > Remove DQMH Event utility."
            # "Do Something Else - Replace this message with functionality for your own application."
            n131 = Variant To Data(error in=w263, type=T10 {"Do Something Else Msg"="", "X"=0.0} ("Do Something Else Argument"), Variant=w258) -> (data=w259:T10, error out=w262:errorcluster)
            n132 = Unbundle By Name(w259) -> ("Do Something Else Msg"=w257:string, "X"=w256:dbl)
            "X" <- w256
            n133 = Format Into String(initial string=w257, w256) -> (resulting string=w255:string)  [unwired: 2 in, 1 out]
            n134 = local write "Status"(w255) -> ()
            n135 = call "Status Updated.vi"("Status"=w255) -> ()  [unwired: 10 in, 1 out]
          }
          frame "Do Something Else and Wait for Reply" {
            w271 = "X(%.2f)+Offset(%.2f)=%.2f"  # status message format string
            # "#DQMH_HowTo The 'Do Something' messages are instructional in nature and can be removed."
            # "Send back X with a random offset"
            # "Do Something Else and Wait for Reply - Replace this message with functionality for your own application. Note that this message must fire a notifier to let callers know it has finished execution, and it returns an error if the 'Value' is negative."
            n136 = Random Number (0-1)() -> (number: 0 to 1=w273:dbl)
            n137 = Variant To Data(error in=w282, type=T11 {"Do Something Else Msg"="", "X"=0.0, "Wait Notifier"=refnum, "wait for reply"=FALSE} ("Do Something Else and Wait for Reply Argument"), Variant=w276) -> (data=w277:T11, error out=w280:errorcluster)
            n138 = Unbundle By Name(w277) -> ("Wait Notifier"=w264:refnum<notifier>, "Do Something Else Msg"=w275:string, "X"=w272:dbl, "wait for reply"=w268:bool)
            n139 = Add(x=w273, y=w272) -> (x+y=w267:dbl)
            n140 = local write "X"(w272) -> ()
            n141 = Less Than 0?(x=w267) -> (x < 0?=w270:bool)
            n142 = Format Into String(format string=w271, initial string=w275, w272, w273, w267) -> (resulting string=w269:string)  [unwired: 1 in, 1 out]
            n143 = case shown="True" w270 {
              tunnel: [_ w289] -> w265
              frame False {
              }
              frame True {
                n144 = xnode "Error Ring"() -> ("error out"=w289:errorcluster)
              }
            }
            n145 = Bundle By Name(cluster=T18 {"Value"=0.0, "error"={"status"=FALSE, "code"=0, "source"=""}} ("notification"), "error"=w265, "Value"=w267) -> (w266:T18)
            n146 = local write "Status"(w269) -> ()
            n147 = call "Status Updated.vi"("Status"=w269) -> ()  [unwired: 10 in, 1 out]
            n148 = case shown="True" w268 {
              tunnel: w266 -> [_ w285]
              tunnel: w264 -> [_ w284]
              frame False {
              }
              frame True {
                # "Simulate an operation that requires a wait."
                n149 = flat-sequence {
                  tunnel: w285 -> [w288]
                  tunnel: w284 -> [w287]
                  tunnel: w283 -> [_]
                  frame #0 {
                    n150 = Send Notification(notification=w288, notifier=w287) -> ()  [unwired: 1 in, 2 out]
                  }
                }
                n151 = Wait (ms)(milliseconds to wait=u32 1000) -> (millisecond timer value=w283:u32)
              }
            }
            n152 = Merge Errors(w280, w265) -> (w281:errorcluster)
          }
          frame "Update control" {
            # "Update control on user panel"
            n153 = Variant To Data(error in=w308, type=T14 {"Filter"=0, "Gain"=0.0, "Bit rate"=0.0, "ISO/IEC w "=enum."14443 Type A", "BI"={"R"=0.0, "C"=0.0, "L"=0.0}, "BM"={"R"=0.0, "C"=0.0, "L"=0.0}, "M"={"Метка"=4, "Считыветель"=4}, "Type noise"=enum."Гауссовский шум", "Link"=enum."UPLINK", "Noise attenuator"=0.0, "Signal gain"=1.0, "Distance"=0.0} ("Sett data"), Variant=w305) -> (data=w304:T14, error out=w306:errorcluster)
            n154 = Unbundle By Name(w304) -> ("ISO/IEC w"=w302:T1, "Gain"=w301:dbl, "Bit rate"=w300:dbl, "Filter"=w299:i32, "Type noise"=w298:T2, "M"=w297:cluster{"Метка":i64, "Считыветель":i64}, "BM"=w296:cluster{"R":dbl, "C":dbl, "L":dbl}, "BI"=w295:cluster{"R":dbl, "C":dbl, "L":dbl})
            n155 = local write "Выбор стандарта"(w302) -> ()
            n156 = local write "Усилитель сигнала"(w301) -> ()
            n157 = local write "Bit rate"(w300) -> ()
            n158 = local write "Filter"(w299) -> ()
            n159 = local write "Type noise w"(w298) -> ()
            n160 = local write "M w"(w297) -> ()
            n161 = local write "BM"(w296) -> ()
            n162 = local write "BI"(w295) -> ()
          }
          frame "---Copy This Frame---" {
            # "Duplicate this frame when creating new messages.  Change this comment in the duplicated frame to describe this message."
            n163 = Merge Errors(w311) -> (w310:errorcluster)
          }
          frame "USER menu" {
            # "Duplicate this frame when creating new messages.  Change this comment in the duplicated frame to describe this message."
            n164 = Variant To Data(error in=w318, type="", Variant=w317) -> (data=w315:string, error out=w314:errorcluster)
            n165 = case shown="\"ANALYS\"" w315 {
              selector: w315 -> [w322 _ _ _ _ _]
              tunnel: w314 -> [w324 w329 w332 w340 w348 w384]
              tunnel: [w323 w328 w331 w339 w368 w384] -> w313
              tunnel: w312 -> [w325 w327 w333 _ _ _]
              frame "DOWN", "UP" {
                n166 = To Variant(anything=w322) -> (Variant=w321:variant)
                n167 = call-poly <vilib>:"Delacor_lib_QMH_Enqueue Message (poly).vi"("error in (no error)"=w324, "Message Data"=w321, "Message"="LINK", "Message Queue in"=w325) -> ("error out"=w323:errorcluster)  [unwired: 6 in, 1 out]
              }
              frame "HELP" {
                n168 = call-poly <vilib>:"Delacor_lib_QMH_Enqueue Message (poly).vi"("error in (no error)"=w329, "Message"="USER help", "Message Queue in"=w327) -> ("error out"=w328:errorcluster)  [unwired: 7 in, 1 out]
              }
              frame "SET" {
                n169 = call-poly <vilib>:"Delacor_lib_QMH_Enqueue Message (poly).vi"("error in (no error)"=w332, "Message"="Set panel", "Message Queue in"=w333) -> ("error out"=w331:errorcluster)  [unwired: 7 in, 1 out]
              }
              frame "POWER" {
                n170 = local read "Link"() -> (w338:T3)
                n171 = Equal?(x=w338, y=Link."UPLINK" ("Link")) -> (x = y?=w336:bool)
                n172 = case shown="True" w336 {
                  tunnel: w340 -> [w342 w344]
                  tunnel: [w341 w344] -> w339
                  tunnel: "Включен канал UPLINK. Анализ питания метки возможен только в режиме канала DOWNLINK. Переключите канал и повторите попытку." ("message") -> [_ w343]
                  frame False {
                    n173 = call "Show Power.vi"("error in (no error)"=w342) -> ("error out"=w341:errorcluster)  [unwired: 10 in]
                  }
                  frame True {
                    n174 = One Button Dialog(message=w343) -> ()  [unwired: 1 in, 1 out]
                  }
                }
              }
              frame "ANALYS" {
                n175 = local read "Иммитатор расстояния"() -> (w345:dbl)
                n176 = local read "Усилитель сигнала"() -> (w358:dbl)
                n177 = local read "Усилитель сигнала"() -> (w346:dbl)
                n178 = property on="Иммитатор расстояния" class="Slide (strict)"() -> ("Scale.Maximum"=w361:dbl)  [unwired: 2 in, 2 out]
                n179 = property on="Аттенюатор шума" class="Knob (strict)"() -> ("Scale.Maximum"=w362:dbl)  [unwired: 2 in, 2 out]
                n180 = local read "Выбор стандарта"() -> (w356:T1)
                n181 = local read "Link"() -> (w367:T3)
                n182 = local read "Type noise w"() -> (w351:T2)
                n183 = local read "Bit rate"() -> (w357:dbl)
                n184 = local read "Filter"() -> (w359:i32)
                n185 = local read "M w"() -> (w353:cluster{"Метка":i64, "Считыветель":i64})
                n186 = local read "BM"() -> (w354:cluster{"R":dbl, "C":dbl, "L":dbl})
                n187 = local read "BI"() -> (w355:cluster{"R":dbl, "C":dbl, "L":dbl})
                n188 = Equal?(x=w367, y=Link."DOWNLINK" ("Link")) -> (x = y?=w365:bool)
                n189 = Bundle(cluster=T19 {"min attenuator"=0.0, "max distanse"=0.0, "num sample"=3.0, "type"=enum."Noise"} ("data"), "min attenuator"=w362, "max distanse"=w361) -> (w349:T19)  [unwired: 2 in]
                n190 = Bundle By Name(cluster=T14 {"Filter"=0, "Gain"=0.0, "Bit rate"=0.0, "ISO/IEC w "=enum."14443 Type A", "BI"={"R"=0.0, "C"=0.0, "L"=0.0}, "BM"={"R"=0.0, "C"=0.0, "L"=0.0}, "M"={"Метка"=4, "Считыветель"=4}, "Type noise"=enum."Гауссовский шум", "Link"=enum."UPLINK", "Noise attenuator"=0.0, "Signal gain"=1.0, "Distance"=0.0} ("Sett data"), "Filter"=w359, "Gain"=w358, "Bit rate"=w357, "ISO/IEC w"=w356, "BI"=w355, "BM"=w354, "M"=w353, "Type noise"=w351, "Distance"=w345, "Noise attenuator"=w346) -> (w352:T14)
                n191 = call "Analys menu.vi"("error in (no error)"=w348, "data in"=w349) -> ("error out"=w347:errorcluster, "close win?"=w364:bool, "data out"=w363:T19)  [unwired: 7 in]
                n192 = case shown="False" w364 {
                  tunnel: [w374 w383] -> w368
                  tunnel: w347 -> [w373 w383]
                  tunnel: w365 -> [w372 _]
                  tunnel: w363 -> [w371 _]
                  tunnel: w352 -> [w370 _]
                  frame False {
                    # "норм настройки"
                    n193 = To Variant(anything=w370) -> (Variant=w369:variant)
                    n194 = case shown="True" w372 {
                      tunnel: [w376 w382] -> w374
                      tunnel: w373 -> [w378 w381]
                      tunnel: w371 -> [w377 w380]
                      tunnel: w369 -> [w375 w379]
                      frame False {
                        n195 = call "Analys.vi"("error in (no error)"=w378, "Data link"=w375, "data"=w377) -> ("error out"=w376:errorcluster)  [unwired: 8 in]
                      }
                      frame True {
                        n196 = call "Analys.vi"("error in (no error)"=w381, "Data link"=w379, "data"=w380) -> ("error out"=w382:errorcluster)  [unwired: 8 in]
                      }
                    }
                  }
                  frame True {
                    # "окно закрыто"
                  }
                }
              }
              frame Default {
              }
            }
            n197 = Merge Errors(w313) -> (w320:errorcluster)
          }
          frame "LINK" {
            # "Duplicate this frame when creating new messages.  Change this comment in the duplicated frame to describe this message."
            n198 = Variant To Data(error in=w397, type="", Variant=w396) -> (data=w386:string, error out=w392:errorcluster)
            n199 = control-ref of="Instrument"() -> (w394:refnum<vi>)
            n200 = invoke class="SubPnl" method="Remove VI"(reference=w394) -> (reference out=w393:refnum<vi>)  [unwired: 2 in, 2 out]
            n201 = Format Into String(format string="Произведено переключение канала на: %s" ("string"), w386) -> (resulting string=w385:string)  [unwired: 2 in, 1 out]
            n202 = local read "Status"() -> (w389:string)
            n203 = case shown="\"UP\"" w386 {
              tunnel: w393 -> [w401 w407]
              tunnel: w392 -> [w403 w406]
              tunnel: [w402 w405] -> w391
              frame "DOWN", Default {
                n204 = call "CH_LINK.vi"("error in (no error)"=w403, "Subpanel Ref"=w401) -> ("error out"=w402:errorcluster)  [unwired: 9 in]
                n205 = local write "Link"(Link."DOWNLINK" ("Link")) -> ()
              }
              frame "UP" {
                n206 = local write "Link"(Link."UPLINK" ("Link")) -> ()
                n207 = call "Ch_LINK.vi"("error in (no error)"=w406, "Subpanel Ref"=w407) -> ("error out"=w405:errorcluster)  [unwired: 9 in]
              }
            }
            n208 = Concatenate Strings(w385, "\r", w389) -> (w390:string)
            n209 = local write "Status"(w390) -> ()
            n210 = Merge Errors(w391) -> (w399:errorcluster)
          }
          frame "USER help" {
            n211 = One Button Dialog(message="Здесь будет помощь для студентов") -> ()  [unwired: 1 in, 1 out]
          }
          frame "Set panel" {
            n212 = call "Show Panel.vi"("error in (no error)"=w412) -> ("error out"=w411:errorcluster)  [unwired: 10 in]
          }
          frame "Update control BC" {
            n213 = Variant To Data(error in=w420, type=T14 {"Filter"=0, "Gain"=0.0, "Bit rate"=0.0, "ISO/IEC w "=enum."14443 Type A", "BI"={"R"=0.0, "C"=0.0, "L"=0.0}, "BM"={"R"=0.0, "C"=0.0, "L"=0.0}, "M"={"Метка"=4, "Считыветель"=4}, "Type noise"=enum."Гауссовский шум", "Link"=enum."UPLINK", "Noise attenuator"=0.0, "Signal gain"=1.0, "Distance"=0.0} ("Sett data"), Variant=w418) -> (data=w416:T14, error out=w419:errorcluster)
            n214 = Unbundle By Name(w416) -> ("ISO/IEC w"=w415:T1, "Gain"=w414:dbl)
            n215 = local write "Выбор стандарта"(w415) -> ()
            n216 = local write "Усилитель сигнала"(w414) -> ()
          }
          frame "Read ini" {
            n217 = Variant To Data(error in=w433, type=ISO."15693" ("NewVal"), Variant=w430) -> (data=w429:T1, error out=w432:errorcluster)
            n218 = Bundle By Name(cluster=T14 {"Filter"=0, "Gain"=0.0, "Bit rate"=0.0, "ISO/IEC w "=enum."14443 Type A", "BI"={"R"=0.0, "C"=0.0, "L"=0.0}, "BM"={"R"=0.0, "C"=0.0, "L"=0.0}, "M"={"Метка"=4, "Считыветель"=4}, "Type noise"=enum."Гауссовский шум", "Link"=enum."UPLINK", "Noise attenuator"=0.0, "Signal gain"=1.0, "Distance"=0.0} ("Sett data"), "ISO/IEC w"=w429) -> (w436:T14)
            n219 = call "Read ini.vi"("error in (no error)"=w432, "Sett data"=w436) -> ("error out"=w434:errorcluster, "Sett data out"=w435:T14)  [unwired: 8 in]
            n220 = Unbundle By Name(w435) -> ("Gain"=w425:dbl, "Bit rate"=w424:dbl, "Filter"=w423:i32, "Type noise"=w422:T2, "M"=w428:cluster{"Метка":i64, "Считыветель":i64}, "BM"=w427:cluster{"R":dbl, "C":dbl, "L":dbl}, "BI"=w426:cluster{"R":dbl, "C":dbl, "L":dbl})
            n221 = local write "Усилитель сигнала"(w425) -> ()
            n222 = local write "Bit rate"(w424) -> ()
            n223 = local write "Filter"(w423) -> ()
            n224 = local write "Type noise w"(w422) -> ()
            n225 = local write "M w"(w428) -> ()
            n226 = local write "BM"(w427) -> ()
            n227 = local write "BI"(w426) -> ()
          }
          frame "--- Exit and Error Handling---" {
            # "Separator - The following cases handle errors and exit messages."
          }
          frame "Simulate MHL Error" {
            # "#DQMH_HowTo The 'Simulate MHL Error' button  illustrates how the MHL handles errors. This event is instructional in nature and can be removed."
            # "Simulate an error occurring at the MHL"
            n228 = call "Module Name--constant.vi"() -> ("Module Name"=w441:string)  [unwired: 11 in]
            n229 = xnode "Error Ring"("parameter 0"=w441) -> ("error out"=w443:errorcluster)
            n230 = Merge Errors(w445, w443) -> (w444:errorcluster)
          }
          frame "Error" {
            # "#CodeRecommended - If you ever change the name of this \"Error\" message, you'll need to update the name in the Check Loop Error.vi as well."
            # "#CodeRecommended - If the module is running in standalone mode (External Launch = FALSE), this code will pop up an error dialog and call the 'Exit' message if an error occurs. Add more fine-grained error handling here."
            # "Error - Check the error message data and respond accordingly. This message is sent by the \"Error Handler\" VIs at the end of each loop in this application."
            n231 = property class="Module Admin"(reference=w454) -> ("Accessors:External Launch"=w453:bool)  [unwired: 1 in, 2 out]
            n232 = Variant To Data(error in=w462, type=errorcluster {"status"=FALSE, "code"=0, "source"=""} ("error constant"), Variant=w456) -> (data=w463:errorcluster, error out=w460:errorcluster)
            n233 = call "Error Reported.vi"("Error"=w463) -> ()  [unwired: 10 in, 1 out]
            n234 = case shown="True" w453 {
              tunnel: [w468 _] -> w459
              tunnel: w455 -> [w466 _]
              tunnel: w463 -> [w467 _]
              frame False {
                # "If the module is running standalone, then pop up an error dialog and call the \"Exit\" message."
                n235 = call <vilib>:"Simple Error Handler.vi"("error in (no error)"=w467) -> ()  [unwired: 4 in, 5 out]
                n236 = call-poly <vilib>:"Delacor_lib_QMH_Enqueue Message (poly).vi"("Priority Message? (F)"=TRUE, "Message"="Exit", "Message Queue in"=w466) -> ("error out"=w468:errorcluster)  [unwired: 7 in, 1 out]
              }
              frame True {
                # "If the module was launched externally, calling the Error Reported broadcast VI is the only action performed by the \"Error\" message. The module's caller can then process the error appropriately."
              }
            }
            n237 = Merge Errors(w460, w459) -> (w458:errorcluster)
            n238 = local write "error out"(w458) -> ()
          }
          frame "Exit" {
            w475 = "Server"
            w474 = TRUE
            w480 = 91  # 91: not all Exit messages will have an argument
            w482 = TRUE  # Stop the VI
            # "Release the message queue reference"
            # "Exit - Exit the application."
            n239 = Variant To Data(error in=w489, type=T13 {"Origin"="", "Exit via Stop Module Req?"=FALSE, "Wait for Module to stop?"=FALSE} ("Stop Argument"), Variant=w481) -> (data=w478:T13, error out=w485:errorcluster)
            n240 = control-ref of="This VI"() -> (w477:refnum<vi>)
            n241 = call "Handle Exit.vi"("Stop Argument"=w478, "Admin in"=w476, "VI reference"=w477) -> ("error out"=w470:errorcluster)  [unwired: 7 in, 1 out]
            n242 = call <vilib>:"Clear Errors.vi"("error in (no error)"=w485, "specific error code to clear (0: all)"=w480) -> ("error out"=w488:errorcluster)  [unwired: 4 in, 1 out]
            n243 = local read "Status"() -> (w473:string)
            n244 = call "Stop Module.vi"("Wait for Module to Stop? (F)"=w474, "Origin"=w475) -> ()  [unwired: 9 in, 1 out]
            n245 = Concatenate Strings("Закрытие приложения" ("string"), "\r", w473) -> (w469:string)
            n246 = call "Stop Module.vi"("Wait for Module to Stop? (F)"=w474, "Origin"=w475) -> ()  [unwired: 9 in, 1 out]
            n247 = call-dynamic "Delacor_lib_QMH_Release Message Queue.vi"("error in (no error)"=w488, "Message Queue"=w484) -> ("error out"=w487:errorcluster)  [unwired: 9 in]
            n248 = call "Log.vi"("Log in"=w469) -> ()  [unwired: 11 in]
            n249 = call "Stop Module.vi"("Wait for Module to Stop? (F)"=w474, "Origin"=w475) -> ()  [unwired: 9 in, 1 out]
            n250 = Merge Errors(w487, w470) -> (w486:errorcluster)
          }
          frame Default {
            # "'Default' case only runs if there is a message that isn't defined in any of the other cases.  Output a programming error."
            n251 = call "Module Name--constant.vi"() -> ("Module Name"=w490:string)  [unwired: 11 in]
            n252 = xnode "Error Ring"("parameter 0"=w491, "parameter 1"=w490) -> ("error out"=w495:errorcluster)
            n253 = Merge Errors(w493, w495) -> (w494:errorcluster)
          }
        }
        n254 = call-dynamic "Delacor_lib_QMH_Error Handler - Message Handling Loop.vi"("error in (no error)"=w221, "Message Queue in"=w211) -> ("dup error in"=w218:errorcluster)  [unwired: 8 in, 1 out]
      }
    }
    frame Error {
      # "Synchronize Caller Events.vi will inform Start Module.vi that the module has launched and will let the code calling Start Module.vi register for broadcasts and would permit the caller receive the broadcast that an error occurred at launch time."
      n255 = call "Synchronize Caller Events.vi"("Singleton Module Admin in"=w504) -> ("error out"=w509:errorcluster)  [unwired: 9 in, 1 out]
      n256 = call "Module Name--constant.vi"() -> ("Module Name"=w507:string)  [unwired: 11 in]
      n257 = Format Into String(format string="An error occurred during initialization. %s is no longer running.", w507) -> (resulting string=w505:string)  [unwired: 2 in, 1 out]
      n258 = Merge Errors(w511, w509) -> (w510:errorcluster)
      n259 = call "Error Reported.vi"("Additional Information"=w505, "Error"=w510) -> ()  [unwired: 9 in, 1 out]
    }
  }
  n260 = Merge Errors(w20, w23) -> (w19:errorcluster)
  n261 = call "Close Module.vi"("error in (no error)"=w19, "Module Admin in"=w15) -> ("error out"=w21:errorcluster, "External Launch"=w8:bool, "Module Admin out"=w9:refnum<class "Delacor_lib_QMH_Module Admin.lvclass">)  [unwired: 7 in]
  n262 = Unregister For Events(event registration refnum=w14, error in=w21) -> (error out=w18:errorcluster)
  "error out" <- w18
  n263 = case "External Launch?" shown="True" w8 {
    tunnel: w18 -> [_ w512]
    frame False {
    }
    frame True {
      n264 = case shown="No Error" w512 {
        frame No Error {
          n265 = invoke class="VI" method="FP.Close"() -> ()  [unwired: 3 in, 3 out]
        }
        frame Error {
          n266 = invoke class="VI" method="FP.Open"("Activate"=TRUE ("Activate?")) -> ()  [unwired: 4 in, 5 out]
        }
      }
    }
  }
  n267 = local write "Module Admin"(w9) -> ()
